vi "1.vi"(8 "Error In":errorcluster) -> (0 "Error Out":errorcluster, 3 "buffer":cluster{"PIPE in":i32, "PIPE OUT":i32})   [LabVIEW 2016]
uses:
  <vilib>/Utility/error.llb/Error Cluster From Error Code.vi
  <vilib>/ErrorRing/Error Ring.xnode
  microchip_solutions_v2013-06-15/USB/Tools/MCHPUSB Custom Driver/Mpusbapi/Dll/Borland_C/Source/mpusbapi.dll
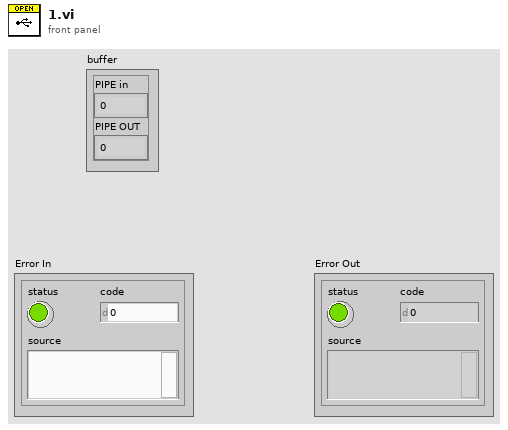
[diagram p1: front panel]
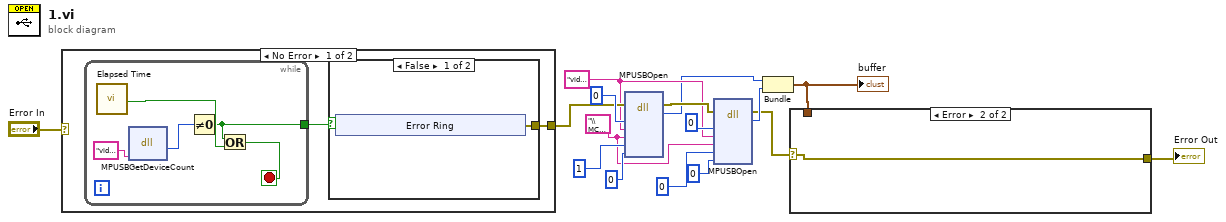
[diagram p0: block diagram]
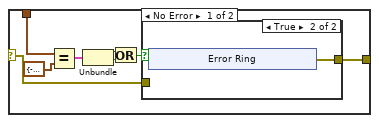
[diagram p2: hidden frame]
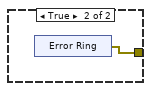
[diagram p4: hidden frame]
diagram:
  w7 = "vid_04d8&pid_000b" ("pVID_PID")
  w6 = "\\MCHP_EP1" ("pEP")
  n1 = case shown="No Error" "Error In" {
    selector: "Error In" -> [_ w32]
    tunnel: [w17 w32] -> w12
    frame No Error {
      n2 = while {
        tunnel: [w27] -> w18
        stop <- w28 stop-if-true
        n3 = call "Elapsed Time"() -> ("Time has Elapsed"=w29:bool)  [unwired: 12 in, 7 out]
        n4 = dll-call lib="C:/microchip_solutions_v2013-06-15/USB/Tools/MCHPUSB Custom Driver/Mpusbapi/Dll/Borland_C/Source/mpusbapi.dll" fn="MPUSBGetDeviceCount"("pVID_PID"="vid_04d8&pid_000b") -> ("N DISPOSITIVOS"=w30:i32)  [unwired: 4 in, 2 out]
        n5 = Not Equal To 0?(x=w30) -> (x != 0?=w27:bool)
        n6 = Or(x=w27, y=w29) -> (x .or. y?=w28:bool)
      }
      n7 = case shown="False" w18 {
        tunnel: [w19 w25] -> w17
        frame False {
          n8 = xnode "Error Ring"() -> ("error out"=w19:errorcluster)
        }
        frame True {
          n9 = xnode "Error Ring"() -> ("error out"=w25:errorcluster)
        }
      }
    }
    frame Error {
    }
  }
  n10 = dll-call lib="C:/microchip_solutions_v2013-06-15/USB/Tools/MCHPUSB Custom Driver/Mpusbapi/Dll/Borland_C/Source/mpusbapi.dll" fn="MPUSBOpen"(error in=w12, "INSTNCIA"=0, "PID_VID"=w7, "pEP"=w6, "dwDIR"=1, "dwReserved"=0) -> (error out=w8:errorcluster, "PIPE"=w5:i32)  [unwired: 7 in, 1 out]
  n11 = dll-call lib="C:/microchip_solutions_v2013-06-15/USB/Tools/MCHPUSB Custom Driver/Mpusbapi/Dll/Borland_C/Source/mpusbapi.dll" fn="MPUSBOpen"(error in=w8, "INSTNCIA"=0, "PID_VID"=w7, "pEP"=w6, "dwDIR"=0, "dwReserved"=0) -> (error out=w3:errorcluster, "PIPE"=w4:i32)  [unwired: 7 in, 1 out]
  n12 = Bundle("PIPE"=w5, "PIPE"=w4) -> (w2:cluster{"PIPE":i32, "PIPE":i32})  [unwired: 1 in]
  "buffer" <- w2
  n13 = case shown="Error" w3 {
    selector: w3 -> [w34 w48]
    tunnel: w2 -> [w40 _]
    tunnel: [w33 w48] -> w1
    frame No Error {
      n14 = Equal?(x=w40, y=cluster{"PIPE":i32, "PIPE":i32} {"PIPE"=-1, "PIPE"=-1}) -> (x = y?=w38:cluster{"PIPE":bool, "PIPE":bool})
      n15 = Unbundle(w38) -> ("PIPE"=w37:bool, "PIPE"=w36:bool)
      n16 = Or(x=w37, y=w36) -> (x .or. y?=w35:bool)
      n17 = case shown="True" w35 {
        tunnel: w34 -> [w41 _]
        tunnel: [w41 w42] -> w33
        frame False {
        }
        frame True {
          n18 = xnode "Error Ring"() -> ("error out"=w42:errorcluster)
        }
      }
    }
    frame Error {
    }
  }
  "Error Out" <- w1
